vi "Memory.Pointer.Bool.Dispose.vi"(8 "error in (no error)":errorcluster, 11 "Bool Pointer":refnum<class "Memory.Pointer.Bool.lvclass">) -> (0 "error out":errorcluster)   [LabVIEW 2016, in "LabVIEW Memory Manager.lvlib" / "Memory.Pointer.Bool.lvclass"]
uses:
  Memory.Pointer.Bool.lvclass
  C:/Users/Ryan/Documents/Git/Sourcetree/LabVIEW-Memory-Manager/Source/Library/Classes/Pointer/Pointer.Void/Memory.Pointer.Void.lvclass
  Pointer.Void/Memory.Pointer.Void.lvclass/Memory.Pointer.Void.ctl
  Pointer.Void/Methods/Memory.Pointer.Get Address.vi
  Pointer.Void/Memory.Pointer.Void.lvclass
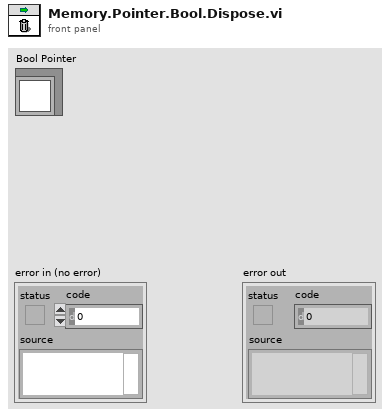
[diagram p1: front panel]
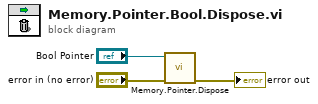
[diagram p0: block diagram]
diagram:
  n1 = call "Memory.Pointer.Dispose.vi"("error in (no error)"="error in (no error)", "Pointer in"="Bool Pointer") -> ("error out"=→"error out":errorcluster)  [unwired: 9 in]
